vi "Register Read Assert Factory.vi"(8 "error in (no error)":errorcluster, 11 "Test Assert Factory":refnum<class "Test Assert Factory.lvclass">) -> (0 "error out":errorcluster, 3 "Test Assert Factory":refnum<class "Test Assert Factory.lvclass">)   [LabVIEW 2020, in "Caraya.lvlib" / "Assert Factory Manager.lvclass"]
doc: "Tries to register an Assert Factory implementation if another implementation is not already registered and returns the currently registered Assert Factory implementation."
uses:
  Assert Factory Manager.lvclass
  Test Assert Factory/Test Assert Factory.lvclass
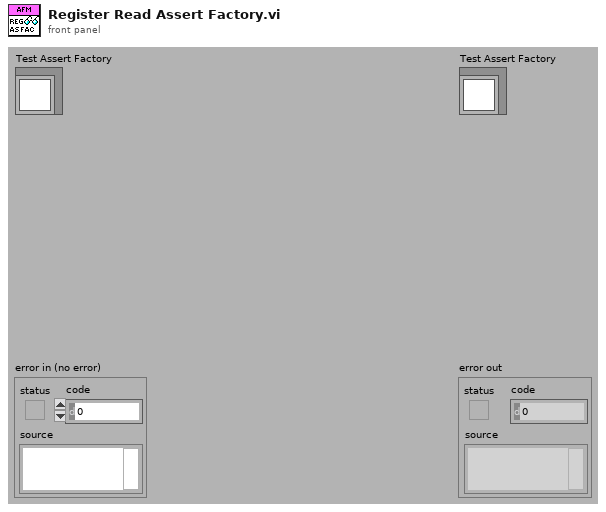
[diagram p1: front panel]
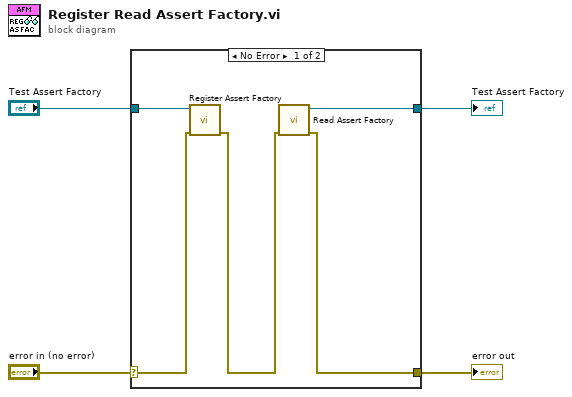
[diagram p0: block diagram]
diagram:
  n1 = case shown="No Error" "error in (no error)" {
    selector: "error in (no error)" -> [w8 w11]
    tunnel: [w6 w11] -> w3
    tunnel: [w5 w10] -> w1
    tunnel: "Test Assert Factory" -> [w9 w10]
    frame No Error {
      n2 = call "Register Assert Factory.vi"("error in (no error)"=w8, "Test Assert Factory"=w9) -> ("error out"=w7:errorcluster)  [unwired: 9 in]
      n3 = call "Read Assert Factory.vi"("error in (no error)"=w7) -> ("error out"=w6:errorcluster, "Test Assert Factory"=w5:refnum<class "Test Assert Factory.lvclass">)  [unwired: 9 in]
    }
    frame Error {
    }
  }
  "error out" <- w3
  "Test Assert Factory" <- w1
